vi "ddsFreqArrayConvert.vi"(7 "Pre 3.0 AOM driver version?":bool, 10 "Register":dbl=4.0 min=0.0 max=15.0 step=1.0 format="%#.6f", 11 "Frequency Array (MHz)":dbl[](array[numeric])=[9.999999978748] min=0.0 max=180.0 step=8.3819e-08 format="%.7f") -> (3 "Characters for FPGA":string="L4071<71<7\r\n")   [LabVIEW 2013, in "DDS9954_v2013.lvlib"]
uses:
  DDS9954_v2013.lvlib
  dataToAscii_32bit.vi
panel:
  out "Original array in U8 format":u8[](array[numeric])
  out "Array from original Code":string[](array[string])
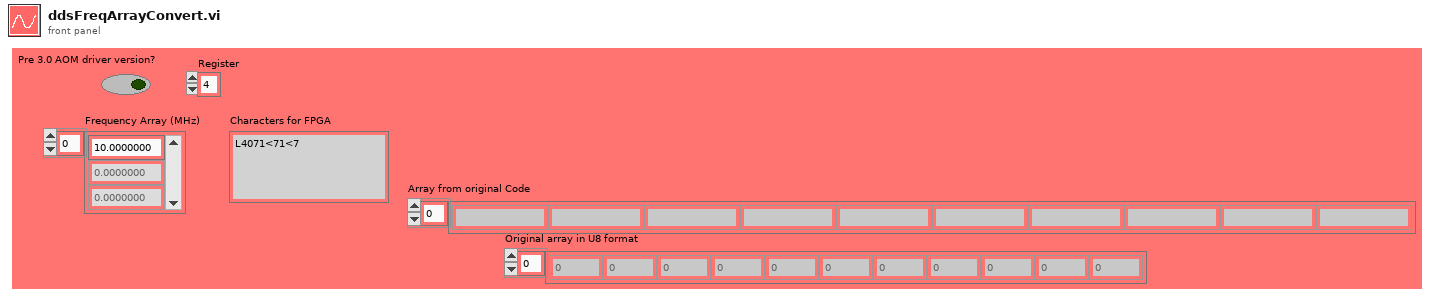
[diagram p1: front panel]
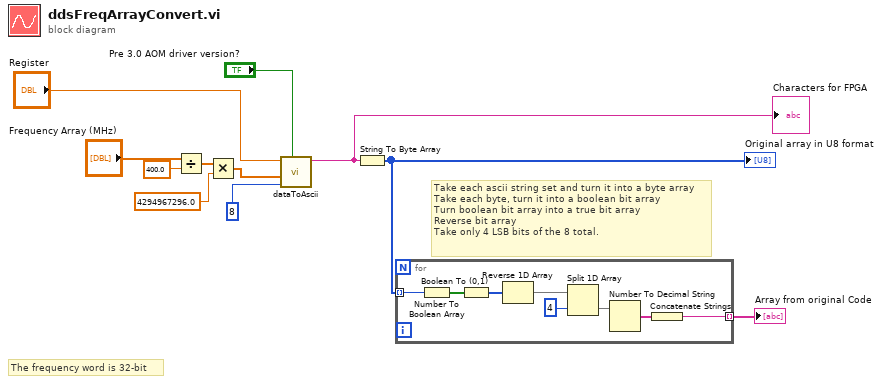
[diagram p0: block diagram]
diagram:
  # "Take each ascii string set and turn it into a byte array\nTake each byte, turn it into a boolean bit array\nTurn boolean bit array into a true bit array\nReverse bit array\nTake only 4 LSB bits of the 8 total."
  # "The frequency word is 32-bit"
  n1 = Divide(x="Frequency Array (MHz)", y=400.0) -> (x/y=w10:dbl[])
  n2 = Multiply(x=w10, y=4294967296.0) -> (x*y=w3:dbl[])
  n3 = call-poly "dataToAscii.vi"("Pre 3.0 AOM driver version?"="Pre 3.0 AOM driver version?", "HEX min width (pre 3.0)"=u8 8, "Input Data"=w3, "Register"="Register") -> ("Characters to FPGA"=w4:string)  [unwired: 7 in]
  "Characters for FPGA" <- w4
  n4 = String To Byte Array(string=w4) -> (unsigned byte array=w7:u8[])
  "Original array in U8 format" <- w7
  n5 = for {
    tunnel: w7 -> [w19] mode=indexing
    tunnel: [w16] -> w6 mode=indexing
    n6 = Number To Boolean Array(number=w19) -> (Boolean array=w18:bool[])
    n7 = Boolean To (0,1)(Boolean=w18) -> (0, 1=w15:i16[])
    n8 = Reverse 1D Array(array=w15) -> (reversed array=w14:i16[])
    n9 = Split 1D Array(array=w14, index=4) -> (second subarray=w12:i16[])  [unwired: 1 out]
    n10 = Number To Decimal String(number=w12) -> (decimal integer string=w17:string[])  [unwired: 1 in]
    n11 = Concatenate Strings(w17) -> (w16:string)
  }
  "Array from original Code" <- w6
